vi "camera shutter.vi"(11 "Array":bool[](array[boolean])) -> (3 "Array 2":bool[](array[boolean]))   [LabVIEW 2014]
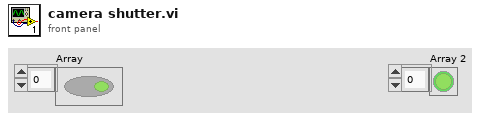
[diagram p1: front panel]
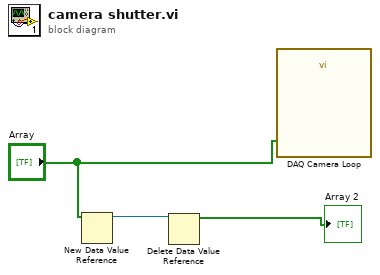
[diagram p0: block diagram]
diagram:
  n1 = New Data Value Reference(data value="Array") -> (data value reference=w3:refnum<data-value>)  [unwired: 1 in, 1 out]
  n2 = Delete Data Value Reference(data value reference=w3) -> (data value=→"Array 2":bool[])  [unwired: 1 in, 1 out]
  n3 = call "DAQ Camera Loop"("data"="Array") -> ()  [unwired: 17 in, 2 out]
